vi "SW_Save_Cluster_to_String.vi"(2 "error in (no error)":errorcluster, 3 "Settings cluster":T1 {"Calibration parameters"."True frame time, s" format="%.10g"; "Calibration parameters"."Disp. calibration info"."Speed, µl per ms" format="%.3g"; "Calibration parameters"."True FPS" format="%.10g"; "Calibration parameters"."Timing calibration sw/hw" format="%.10g"; "Conditions presets array"."Specifier(s)"."Validity criteria(s)"."Validity value" min=0.0 step=0.1 format="%.2g"; "Conditions presets array"."Specifier(s)"."Value" step=1.0 format="%#.2g"; "Recording and saving"."Data post-processing"."Order" min=3 max=11 step=2; "Recording and saving"."Data post-processing"."Length" min=5 max=301 step=2; "Geometry"."Cage type" items=["Round", "Square", "Donut-maze", "T-maze", "Sociability maze", ""]}) -> (0 "error out":errorcluster, 1 "Data String out":string)   [LabVIEW 2018, in "Tracker.lvlib"]
uses:
  Tracker.lvlib
  Controls/CTL_Settings_cluster.ctl
  Controls/CTL_Histogram_parameters.ctl
  Controls/CTL_Filter_selector.ctl
  Controls/CTL_Acquisition_speed_selector.ctl
  Controls/CTL_Segmented_plot_parameters_2.ctl
  Libraries/Cage Diagram/Typedefs/CTL_Cage_type.ctl
  Controls/CTL_Cage_all_segmentation_params_set.ctl
  Controls/CTL_IO_params_cluster.ctl
  Controls/CTL_Conditions_Array.ctl
  Controls/CTL_Conditions_Cluster.ctl
  Controls/CTL_Condition_type.ctl
  Controls/CTL_Comparison_type.ctl
  Controls/CTL_Validity_check_criteria.ctl
  Controls/CTL_Response_info.ctl
  Controls/CTL_Condition_response_type.ctl
  Controls/CTL_Reponse_port_info.ctl
  Controls/CTL_Calibration_parameters.ctl
  Controls/CTL_Dispenser_calibration_info.ctl
  Common_Resources.lvlib
  Libraries/Cage Diagram/Cage Diagram.lvlib
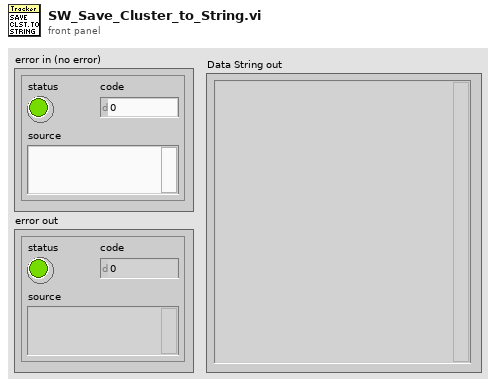
[diagram p1: front panel]
types:
  T1 = typedef "Common_Resources.lvlib/CTL_Settings_cluster.ctl" = cluster{"Defaults":cluster{"Default User":dbl, "VISA Resource Name ":string, "Histogram parameters":T2}, "Recording and saving":cluster{"Researcher name":string, "Name prefix":string, "Data post-processing":T3, "Stop at":dbl, "\"Stop at\" enabled":bool, "Default save folder path":path, "Acquisition FPS":T4}, "Geometry":T5, "IO parameters":T8, "Conditions presets array":T9, "Calibration parameters":T17, "Settings loaded OK":bool}
  T2 = typedef "Common_Resources.lvlib/CTL_Histogram_parameters.ctl" = cluster{"max":dbl, "min":dbl, "# bins":i32, "threshold":dbl, "thr. type":enum16{"higher accepted", "lower accepted"}}
  T3 = typedef "Common_Resources.lvlib/CTL_Filter_selector.ctl" = cluster{"Filter type":enum16{"None", "Savitzky-Golay"}, "Length":i32, "Order":i32}
  T4 = typedef "Common_Resources.lvlib/CTL_Acquisition_speed_selector.ctl" = enum16{"Max", "Optimal", "Eco"}
  T5 = typedef "Common_Resources.lvlib/CTL_Segmented_plot_parameters_2.ctl" = cluster{"Sensor board size":enum16{"", "Large"}, "Bridge swap":bool, "Twisted neck":bool, "Bridge H. offset":sgl, "Bridge V. offset":sgl, "Magnets orientation":sgl, "Cage type":T6, "Cage parameters":T7}
  T6 = typedef "Cage Diagram.lvlib/CTL_Cage_type.ctl" = u16
  T7 = typedef "Common_Resources.lvlib/CTL_Cage_all_segmentation_params_set.ctl" = cluster{"Round":variant, "Square":variant, "Donut-maze":variant, "T-maze":variant, "Sociability-maze":variant}
  T8 = typedef "Common_Resources.lvlib/CTL_IO_params_cluster.ctl" = cluster{"IO general config.":u16, "IO 1 configuration":u16, "IO 2 configuration":u16, "IO 3 configuration":u16, "IO 4 configuration":u16, "Activate ext. RS-232":u16, "IO inversion config.":u16, "Sync capability":u8}
  T9 = typedef "Common_Resources.lvlib/CTL_Conditions_Array.ctl" = T10[]
  T10 = typedef "Common_Resources.lvlib/CTL_Conditions_Cluster.ctl" = cluster{"Enabled":bool, "Name":string, "Specifier(s)":cluster{"Specifier enabled":bool, "Condition type":T11, "Comparison type":T12, "Value":dbl, "Validity criteria(s)":cluster{"V. check enabled":bool, "Criteria":T13, "Validity value":dbl}[]}[], "Response":T14, "Has been set":bool}
  T11 = typedef "Common_Resources.lvlib/CTL_Condition_type.ctl" = enum16{"Speed", "Zone", "Angle to wall"}
  T12 = typedef "Common_Resources.lvlib/CTL_Comparison_type.ctl" = enum16{"Less", "Less or Equal", "Equal", "Greater or Equal", "Greater", "Not Equal"}
  T13 = typedef "Common_Resources.lvlib/CTL_Validity_check_criteria.ctl" = enum16{"Running bout (seconds)", "Running bout (meters)"}
  T14 = typedef "Common_Resources.lvlib/CTL_Response_info.ctl" = cluster{"Response type":T15, "TTL port":T16, "TTL pulse length, ms":dbl}
  T15 = typedef "Common_Resources.lvlib/CTL_Condition_response_type.ctl" = enum16{"None", "Air puff", "Liquid reward", "TTL pulse", "TTL pulse (ubr)", "TTL signal"}
  T16 = typedef "Common_Resources.lvlib/CTL_Reponse_port_info.ctl" = enum16{"Port 1", "Port 2", "Port 3", "Port 4"}
  T17 = typedef "Common_Resources.lvlib/CTL_Calibration_parameters.ctl" = cluster{"Timing calibration sw/hw":dbl, "True FPS":dbl, "True frame time, s":dbl, "Disp. calibration info":T18}
  T18 = typedef "Common_Resources.lvlib/CTL_Dispenser_calibration_info.ctl" = cluster{"Channel":u8, "Speed, µl per ms":dbl}[]
  T19 = cluster{"Default User":dbl, "VISA Resource Name ":string, "Histogram parameters":T2}
  T20 = cluster{"Researcher name":string, "Name prefix":string, "Data post-processing":T3, "Stop at":dbl, "\"Stop at\" enabled":bool, "Default save folder path":path, "Acquisition FPS":T4}
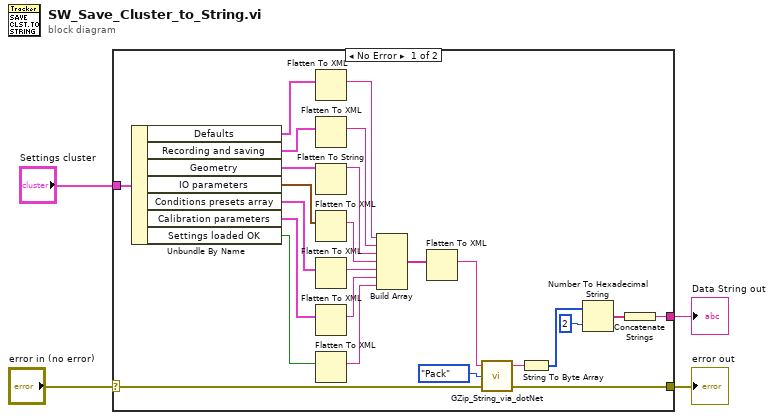
[diagram p0: block diagram]
diagram:
  n1 = case shown="No Error" "error in (no error)" {
    selector: "error in (no error)" -> [w12 w30]
    tunnel: "Settings cluster" -> [w15 _]
    tunnel: [w5 _] -> w2
    tunnel: [w11 w30] -> w1
    frame No Error {
      n2 = Unbundle By Name(w15) -> ("Defaults"=w23:T19, "Recording and saving"=w24:T20, "Geometry"=w25:T5, "IO parameters"=w26:T8, "Conditions presets array"=w27:T9, "Calibration parameters"=w28:T17, "Settings loaded OK"=w29:bool)
      n3 = Flatten To XML(anything=w23) -> (xml string=w16:string)
      n4 = Flatten To XML(anything=w24) -> (xml string=w17:string)
      n5 = Flatten To String(anything=w25) -> (data string=w18:string)  [unwired: 3 in, 2 out]
      n6 = Flatten To XML(anything=w26) -> (xml string=w19:string)
      n7 = Flatten To XML(anything=w27) -> (xml string=w20:string)
      n8 = Flatten To XML(anything=w28) -> (xml string=w21:string)
      n9 = Flatten To XML(anything=w29) -> (xml string=w22:string)
      n10 = Build Array(w16, w17, w18, w19, w20, w21, w22) -> (w14:string[])
      n11 = Flatten To XML(anything=w14) -> (xml string=w13:string)
      n12 = call "GZip_String_via_dotNet.vi"("error in (no error)"=w12, "Action"=enum16{"Pack", "Unpack"}."Pack", "String Input"=w13) -> ("error out"=w11:errorcluster, "String Output (GZipped/UnGZipped)"=w6:string)  [unwired: 1 out]
      n13 = String To Byte Array(string=w6) -> (unsigned byte array=w9:u8[])
      n14 = Number To Hexadecimal String(1:i16 2 ("width (-)"), 2:w9) -> (0:w7:string[])
      n15 = Concatenate Strings(w7) -> (w5:string)
    }
    frame Error {
    }
  }
  "Data String out" <- w2
  "error out" <- w1
